vi "Target Logging.vi"(6 "rt fifo":refnum<k33>) -> (0 "Stop Loop":bool)   [LabVIEW 2018]
uses:
  Target Logging Cluster.ctl
  Logging Data Cluster.ctl
  Target Logging Control Signals.ctl
  Target Logging Sensors.ctl
  Sensor Data.ctl
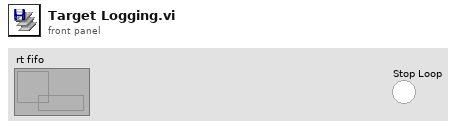
[diagram p1: front panel]
types:
  T1 = enum16{"Idle", "Accumulate", "Write Main", "Write Metadata"}
  T2 = typedef "Target Logging Cluster.ctl" = cluster{"Valid for Logging?":bool, "Data":T3}
  T3 = typedef "Logging Data Cluster.ctl" = cluster{"Control Signals":T4, "Target Sensors":T5}
  T4 = typedef "Target Logging Control Signals.ctl" = cluster{"Phi":dbl, "Gait %":dbl, "ILC Desired Ankle Angle":dbl, "Desired Motor Current":dbl, "Transmission Ratio":dbl, "Passive Torque Estimate":dbl, "Torque Reference":dbl, "Left HS?":bool, "Left HS State":u32, "Right HS?":bool, "Right HS State":u32, "dGRF L":dbl, "dGRF R":dbl, "GRF L (filt) ":dbl, "GRF R (filt)":dbl}
  T5 = typedef "Target Logging Sensors.ctl" = cluster{"Sensors":T6}
  T6 = typedef "Sensor Data.ctl" = cluster{"Motor Current":dbl, "Motor Velocity":dbl, "Ankle Encoder Angle":dbl, "GRF L":dbl, "GRF R":dbl, "Index pulse?":bool, "Roll":dbl, "Pitch":dbl, "Yaw":dbl, "Thigh Angle":dbl}
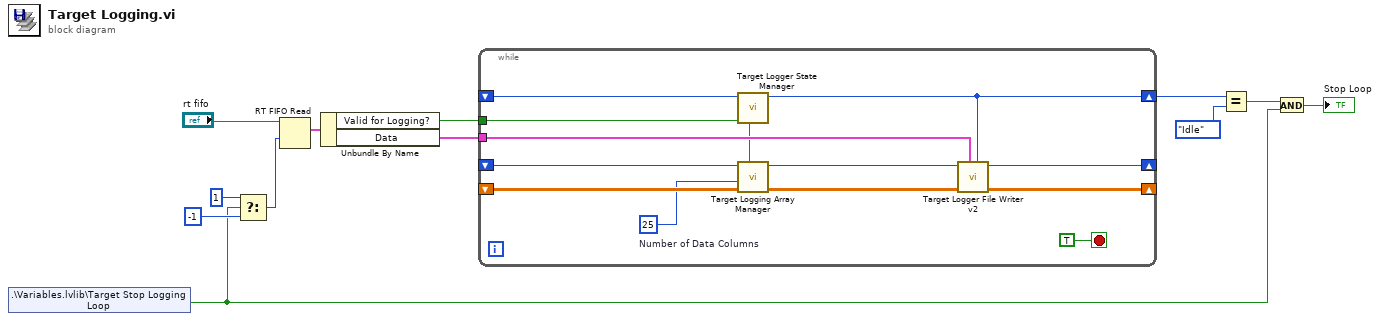
[diagram p0: block diagram]
diagram:
  n1 = shared-variable ".\\Variables.lvlib\\Target Stop Logging Loop"() -> (w1:bool)  [unwired: 1 in, 1 out]
  n2 = Select(t=1, s=w1, f=-1) -> (s? t:f=w10:i32)
  n3 = RT FIFO Read(0:"rt fifo", 2:w10) -> (9:w4:T2)  [unwired: 2 in, 4 out]
  n4 = Unbundle By Name(w4) -> ("Valid for Logging?"=w3:bool, "Data"=w2:T3)
  n5 = while {
    tunnel: w3 -> [w23]
    shift-right: [w16] -> w8
    shift-left: _ -> [w24]
    shift-right: [w21] -> _
    shift-left: _ -> [w19]
    shift-right: [w17] -> _
    shift-left: _ -> [w22]
    tunnel: w2 -> [w15]
    stop <- TRUE stop-if-true
    w18 = 25  # Number of Data Columns
    n6 = call "Target Logger State Manager.vi"("Valid for Logging?"=w23, "Previous State"=w24) -> ("Current State"=w16:T1, "Preallocate Array?"=w13:bool)  [unwired: 8 in]
    n7 = call "Target Logging Array Manager.vi"("Allocate New Array"=w13, "Input Array"=w19, "Number of Data Columns"=w18, "Previous Index"=w22) -> ("Output Array"=w20:dbl[][], "Array Index to Write"=w14:i32)  [unwired: 6 in]
    n8 = call "Target Logger File Writer v2.vi"("State"=w16, "Data"=w15, "Input Array"=w20, "Array Index"=w14) -> ("Output Array"=w21:dbl[][], "Array Index Out"=w17:i32)  [unwired: 6 in]
  }
  n9 = Equal?(x=w8, y=T1."Idle") -> (x = y?=w9:bool)
  n10 = And(x=w9, y=w1) -> (x .and. y?=→"Stop Loop":bool)
